vi "Classification.vi"(1 "Numeric":dbl) -> (0 "Detected Wave":string)   [LabVIEW 2023]
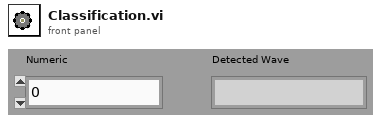
[diagram p1: front panel]
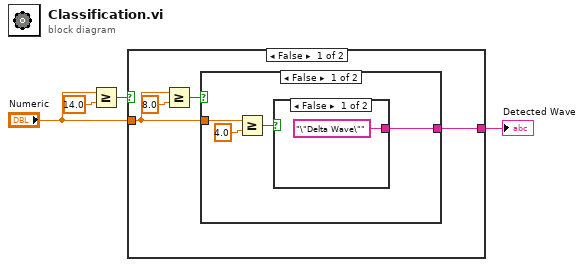
[diagram p0: block diagram]
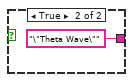
[diagram p2: hidden frame]
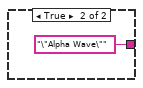
[diagram p3: hidden frame]
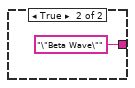
[diagram p4: hidden frame]
diagram:
  n1 = Greater Or Equal?(x="Numeric", y=14.0) -> (x >= y?=w3:bool)
  n2 = case shown="False" w3 {
    tunnel: [w6 "\"Beta Wave\""] -> w4
    tunnel: "Numeric" -> [w5 _]
    frame False {
      n3 = Greater Or Equal?(x=w5, y=8.0) -> (x >= y?=w7:bool)
      n4 = case shown="False" w7 {
        tunnel: [w9 "\"Alpha Wave\""] -> w6
        tunnel: w5 -> [w11 _]
        frame False {
          n5 = Greater Or Equal?(x=w11, y=4.0) -> (x >= y?=w12:bool)
          n6 = case shown="False" w12 {
            tunnel: ["\"Delta Wave\"" "\"Theta Wave\""] -> w9
            frame False {
            }
            frame True {
            }
          }
        }
        frame True {
        }
      }
    }
    frame True {
    }
  }
  "Detected Wave" <- w4
